vi "Controllers_PIDZPositionNoWhile-Archived-2024-01-24.vi"(0 "Task In":refnum<k21>, 1 "SP Femto":dbl=0.1, 2 "Loop Time In":i32, 3 "Piezo In / V":dbl format="%.3g", 5 "Error In":errorcluster, 6 "Alpha":dbl=nan format="%.2f", 7 "DC Bias":dbl=0.2, 8 "Beta":dbl=1.0, 9 "PID gains":T1 {"derivative time (Td, min)" format="%.6f"; "integral time (Ti, min)" format="%.6f"; "proportional gain (Kc)" format="%.6f"}, 10 "Iterator In":i32, 11 "Real time Femto / V":dbl=0.10000000000000014) -> (14 "Task Out":refnum<k21>, 15 "Stop?":bool, 16 "Loop Time Out":u32, 17 "Piezo Out / V":dbl format="%.6g", 18 "Runtime / s":dbl, 19 "Error Out":errorcluster)   [LabVIEW 2023]
uses:
  <vilib>/DAQmx/write.llb/DAQmx Write (Analog 1D DBL NChan 1Samp).vi
  <vilib>/addons/control/pid/pid.llb/PID Advanced (DBL).vi
  <vilib>/DAQmx/miscellaneous.llb/DAQmx Fill In Error Info.vi
  <vilib>/addons/control/pid/NI_PID_pid.lvlib
panel:
  in  "Aquisition Rate (20000) / Hz":dbl
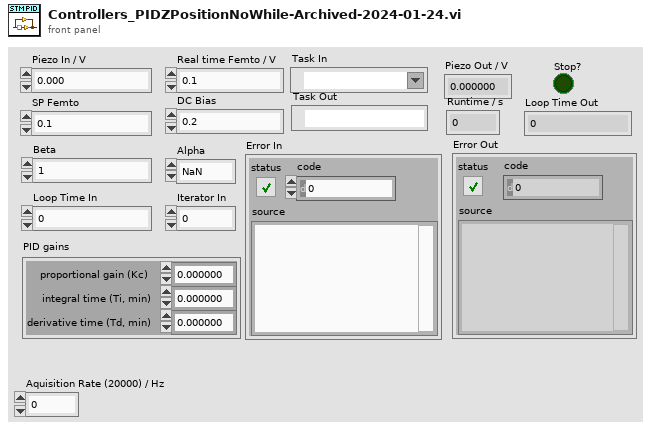
[diagram p1: front panel]
types:
  T1 = cluster{"proportional gain (Kc)":dbl, "integral time (Ti, min)":dbl, "derivative time (Td, min)":dbl}
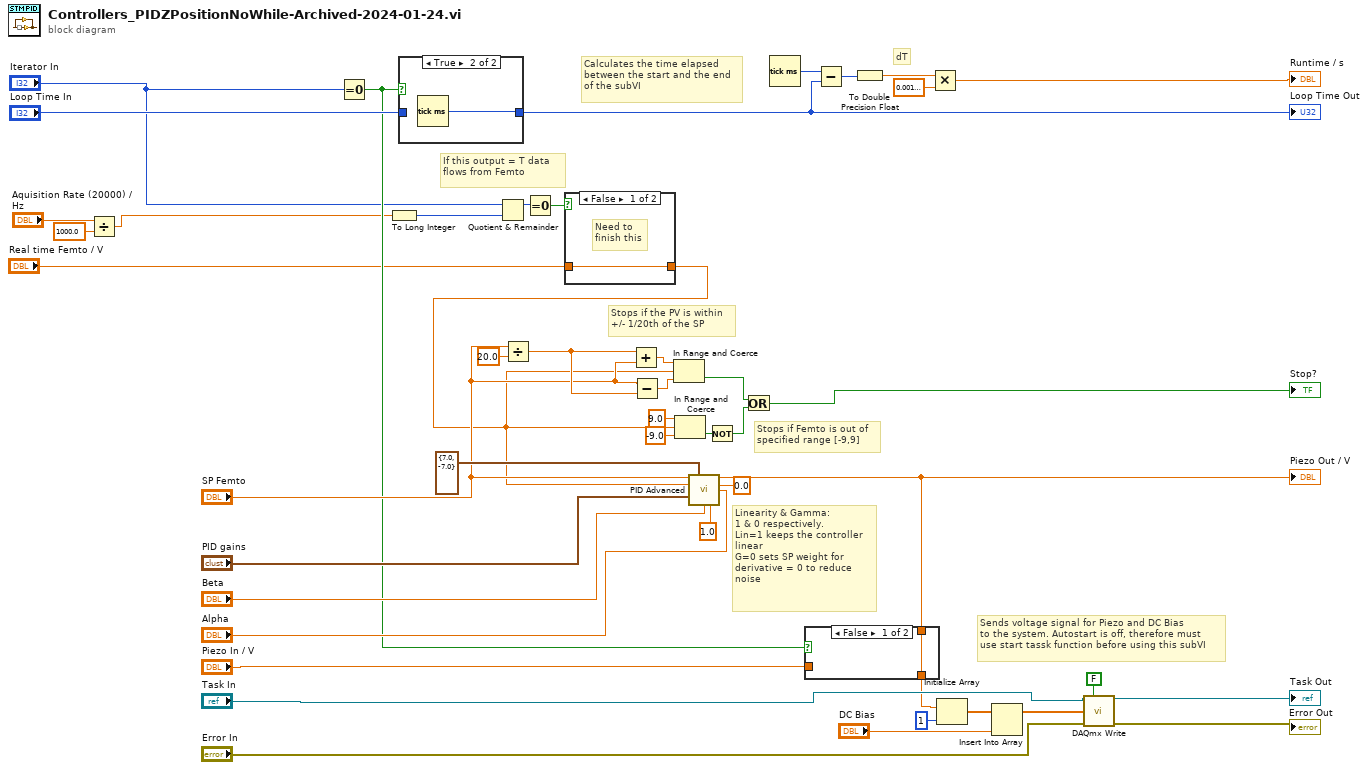
[diagram p0: block diagram]
diagram:
  # "If this output = T data flows from Femto"
  # "Stops if Femto is out of\nspecified range [-9,9]"
  # "Linearity & Gamma:\n1 & 0 respectively.\nLin=1 keeps the controller \nlinear\nG=0 sets SP weight for \nderivative = 0 to reduce\nnoise"
  # "Calculates the time elapsed\nbetween the start and the end\nof the subVI"
  # "Sends voltage signal for Piezo and DC Bias\nto the system. Autostart is off, therefore must\nuse start tassk function before using this subVI"
  # "Stops if the PV is within\n+/- 1/20th of the SP"
  # "dT"
  n1 = Divide(x="Aquisition Rate (20000) / Hz", y=1000.0) -> (x/y=w6:dbl)
  n2 = Equal To 0?(x="Iterator In") -> (x = 0?=w10:bool)
  n3 = To Long Integer(number=w6) -> (32bit integer=w5:i32)
  n4 = case shown="True" w10 {
    tunnel: [w47 w48] -> w29
    tunnel: "Loop Time In" -> [w47 _]
    frame False {
    }
    frame True {
      n5 = Tick Count (ms)() -> (millisecond timer value=w48:u32)
    }
  }
  "Loop Time Out" <- w29
  n6 = Quotient & Remainder(x="Iterator In", y=w5) -> (x-y*floor(x/y)=w4:i32)  [unwired: 1 out]
  n7 = Divide(x="SP Femto", y=20.0) -> (x/y=w21:dbl)
  n8 = Equal To 0?(x=w4) -> (x = 0?=w3:bool)
  n9 = case shown="False" w3 {
    tunnel: "Real time Femto / V" -> [w49 w50]
    tunnel: [w49 w50] -> w1
    frame False {
      # "Need to\nfinish this"
    }
    frame True {
    }
  }
  n10 = Add(x=w21, y="SP Femto") -> (x+y=w23:dbl)
  n11 = Subtract(x="SP Femto", y=w21) -> (x-y=w22:dbl)
  n12 = In Range and Coerce(upper limit=w23, x=w1, lower limit=w22) -> (In Range?=w16:bool)  [unwired: 1 out]
  n13 = In Range and Coerce(upper limit=9.0, x=w1, lower limit=-9.0) -> (In Range?=w20:bool)  [unwired: 1 out]
  n14 = call-poly <vilib>:"PID Advanced.vi"("setpoint"="SP Femto", "output range"=cluster{"output high":dbl, "output low":dbl} {"output high"=7.0, "output low"=-7.0}, "process variable"=w1, "gamma"=0.0, "alpha"="Alpha", "PID gains"="PID gains", "beta"="Beta", "linearity"=1.0) -> ("output"=w13:dbl)  [unwired: 6 in, 1 out]
  "Piezo Out / V" <- w13
  n15 = Not(x=w20) -> (.not. x?=w17:bool)
  n16 = Or(x=w16, y=w17) -> (x .or. y?=→"Stop?":bool)
  n17 = Tick Count (ms)() -> (millisecond timer value=w30:u32)
  n18 = case shown="False" w10 {
    tunnel: w13 -> [w51 _]
    tunnel: [w51 w52] -> w12
    tunnel: "Piezo In / V" -> [_ w52]
    frame False {
    }
    frame True {
    }
  }
  n19 = Subtract(x=w30, y=w29) -> (x-y=w26:u32)
  n20 = To Double Precision Float(number=w26) -> (double precision float=w28:dbl)
  n21 = Multiply(x=w28, y=0.0010000000474974513) -> (x*y=→"Runtime / s":dbl)
  n22 = Initialize Array(w12, 1 ("dimension size")) -> (w35:dbl[])
  n23 = Insert Into Array(array=w35, new element="DC Bias") -> (w34:dbl[])  [unwired: 1 in]
  n24 = call-poly <vilib>:"DAQmx Write.vi"("task/channels in"="Task In", "auto start"=FALSE, "data"=w34, "error in"="Error In") -> ("task out"=→"Task Out":refnum<k21>, "error out"=→"Error Out":errorcluster)  [unwired: 9 in, 1 out]
